vi "Forebrain Main.vi"(8 "error in":errorcluster, 9 "QueueRef":T2, 10 "Mission Notifiers":T1, 11 "NotifierReff":T3) -> (0 "error out":errorcluster)   [LabVIEW 2013]
uses:
  Data/TypeDefs/Notifiers.ctl
  Data/TypeDefs/UTM Location.ctl
  Data/TypeDefs/Sail Set Suggestions.ctl
  Data/TypeDefs/Rudder Set Suggestions.ctl
  Data/TypeDefs/OverrideInformation.ctl
  Data/TypeDefs/OverrideMode.ctl
  Data/TypeDefs/MotorSetup.ctl
  Data/TypeDefs/DynamixelSetupInfo.ctl
  Data/TypeDefs/AirmarStatus.ctl
  Data/TypeDefs/HardwareOnline.ctl
  Data/TypeDefs/DynamixelCycleTracker.ctl
  Data/TypeDefs/RC Input Values.ctl
  Classes/Waypoint/Waypoint.lvclass
  Data/TypeDefs/Queues.ctl
  Data/TypeDefs/MissionNotifiers.ctl
  Classes/Missions/GenericMission/GenericMission.lvclass
  Classes/Obstacle/Obstacle.lvclass
  RIO-OCU_Comm/NetworkStreams/Reader/NetworkStreamReader.lvclass
  RIO-OCU_Comm/NetworkStreams/Writer/NetworkStreamWriter.lvclass
panel:
  out "Number of sailing points added":i32
  out "Added sailing points?":bool
  out "Added intermediate point?":bool
  out "Forebrain Sense Counter":i32
  out "Forebrain Act Loop Counter":i32
  out "Forebrain Think Loop Counter":i32
  out "Connected to OCU?":bool
  # "Debug"
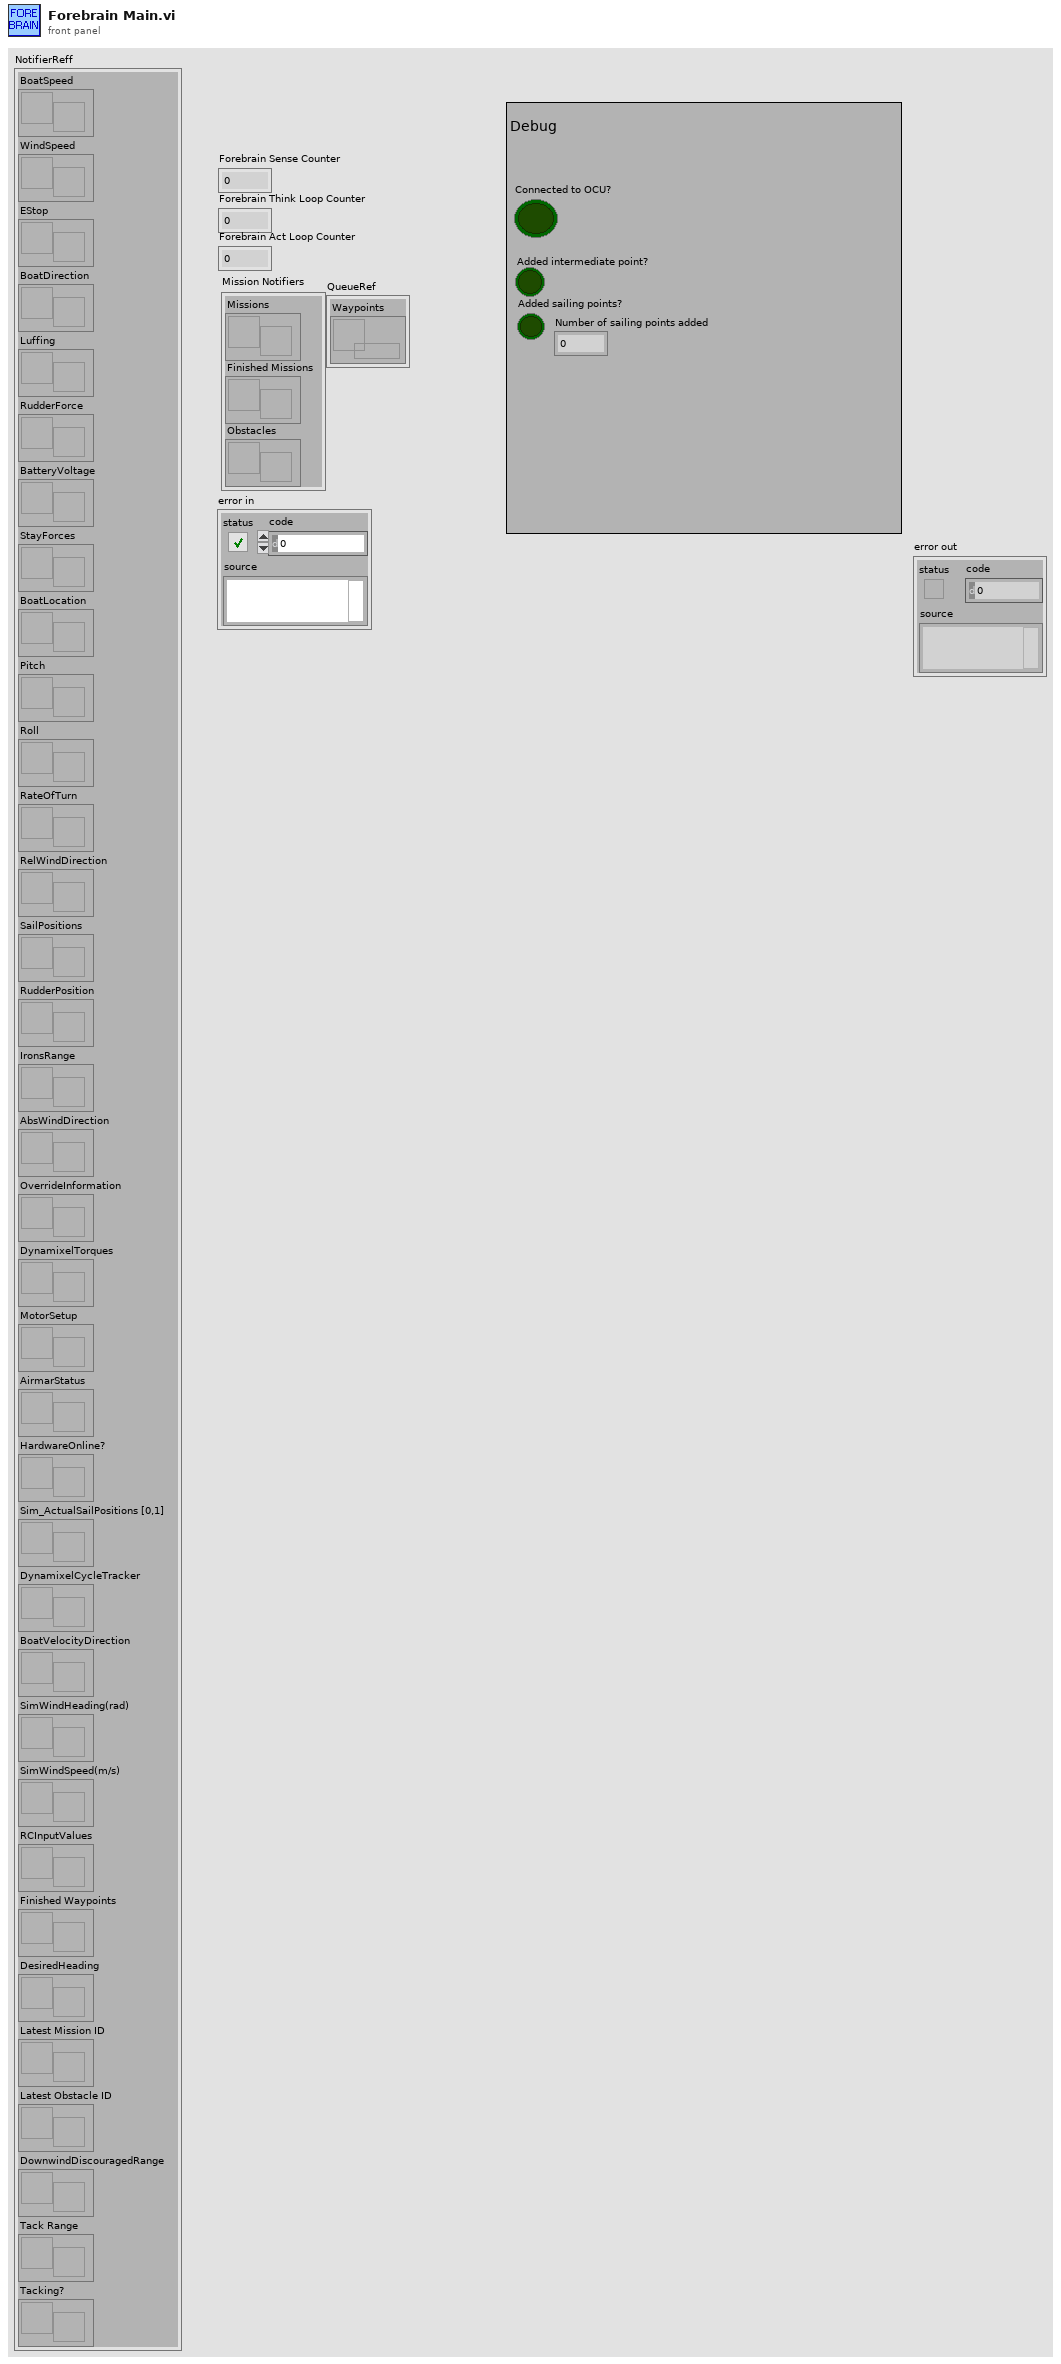
[diagram p1: front panel]
types:
  T1 = typedef "MissionNotifiers.ctl" = cluster{"Missions":refnum<notifier>, "Finished Missions":refnum<notifier>, "Obstacles":refnum<notifier>}
  T2 = typedef "Queues.ctl" = cluster{"Waypoints":refnum<queue>}
  T3 = typedef "Notifiers.ctl" = cluster{"BoatSpeed":refnum<notifier>, "WindSpeed":refnum<notifier>, "EStop":refnum<notifier>, "BoatDirection":refnum<notifier>, "Luffing":refnum<notifier>, "RudderForce":refnum<notifier>, "BatteryVoltage":refnum<notifier>, "StayForces":refnum<notifier>, "BoatLocation":refnum<notifier>, "Pitch":refnum<notifier>, "Roll":refnum<notifier>, "RateOfTurn":refnum<notifier>, "RelWindDirection":refnum<notifier>, "SailPositions":refnum<notifier>, "RudderPosition":refnum<notifier>, "IronsRange":refnum<notifier>, "AbsWindDirection":refnum<notifier>, "OverrideInformation":refnum<notifier>, "DynamixelTorques":refnum<notifier>, "MotorSetup":refnum<notifier>, "AirmarStatus":refnum<notifier>, "HardwareOnline?":refnum<notifier>, "Sim_ActualSailPositions [0,1]":refnum<notifier>, "DynamixelCycleTracker":refnum<notifier>, "BoatVelocityDirection":refnum<notifier>, "SimWindHeading(rad)":refnum<notifier>, "SimWindSpeed(m/s)":refnum<notifier>, "RCInputValues":refnum<notifier>, "Finished Waypoints":refnum<notifier>, "DesiredHeading":refnum<notifier>, "Latest Mission ID":refnum<notifier>, "Latest Obstacle ID":refnum<notifier>, "DownwindDiscouragedRange":refnum<notifier>, "Tack Range":refnum<notifier>, "Tacking?":refnum<notifier>}
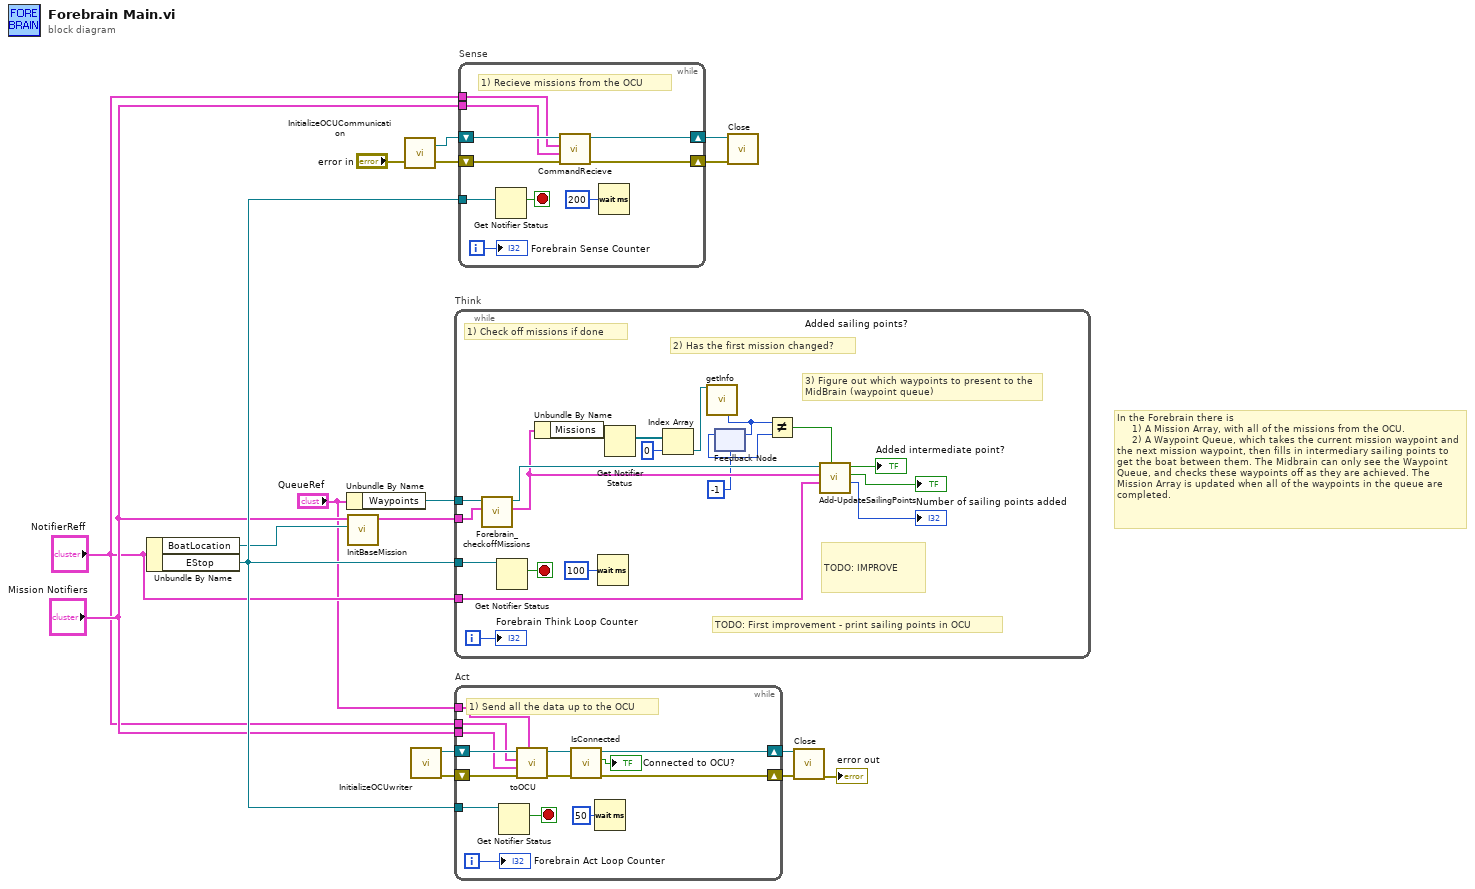
[diagram p0: block diagram]
diagram:
  # "In the Forebrain there is\n     1) A Mission Array, with all of the missions from the OCU.\n     2) A Waypoint Queue, which takes the current mission waypoint and the next mission waypoint, then fills in intermediary sailing points to get the boat between them. The Midbrain can only see the Waypoint Queue, and checks these waypoints off as they are achieved. The Mission Array is updated when all of the waypoints in the queue are completed."
  n1 = Unbundle By Name("NotifierReff") -> ("BoatLocation"=w5:refnum<notifier>, "EStop"=w11:refnum<notifier>)
  n2 = Unbundle By Name("QueueRef") -> ("Waypoints"=w17:refnum<queue>)
  n3 = call "InitBaseMission.vi"("Boat Location"=w5, "Mission Notifiers"="Mission Notifiers") -> ("Mission Notifiers OUT"=w3:T1)  [unwired: 9 in]
  n4 = call "InitializeOCUCommunication.vi"("error in (no error)"="error in") -> ("error out"=w16:errorcluster, "NetworkStreamReader out"=w15:refnum<class "NetworkStreamReader.lvclass">)  [unwired: 1 in]
  n5 = call "InitializeOCUwriter.vi"() -> ("error out"=w8:errorcluster, "NetworkStreamWriter out"=w10:refnum<class "NetworkStreamWriter.lvclass">)  [unwired: 10 in]
  n6 = while "Think" {
    tunnel: w11 -> [w36]
    tunnel: w17 -> [w32]
    tunnel: w3 -> [w33]
    tunnel: "NotifierReff" -> [w21]
    i -> [w34]
    stop <- w37 stop-if-true
    # "TODO: First improvement - print sailing points in OCU"
    # "2) Has the first mission changed?"
    # "TODO: IMPROVE"
    # "3) Figure out which waypoints to present to the MidBrain (waypoint queue)"
    # "1) Check off missions if done"
    n7 = call "Forebrain_checkoffMissions.vi"("Mission Notifiers"=w33, "Waypoints"=w32) -> ("Mission Notifiers OUT"=w30:T1, "Waypoints out"=w31:refnum<queue>)  [unwired: 7 in, 1 out]
    n8 = Get Notifier Status(notifier=w36) -> (current notification=w37:bool)  [unwired: 1 in, 4 out]
    n9 = Unbundle By Name(w30) -> ("Missions"=w29:refnum<notifier>)
    n10 = Wait (ms)(milliseconds to wait=u32 100) -> ()  [unwired: 1 out]
    n11 = Get Notifier Status(notifier=w29) -> (current notification=w28:refnum<class "GenericMission.lvclass">[])  [unwired: 1 in, 4 out]
    n12 = Index Array(array=w28, index=0) -> (element=w26:refnum<class "GenericMission.lvclass">)
    n13 = call-dynamic "getInfo.vi"("GenericMission in"=w26) -> ("ID#"=w25:i16)  [unwired: 6 in, 8 out]
    n14 = feedback-in #1(w25) -> ()
    n15 = feedback #1(i16 -1 ("ID#")) -> (w24:i16)
    n16 = Not Equal?(x=w25, y=w24) -> (x != y?=w22:bool)
    n17 = call "Add-UpdateSailingPoints.vi"("Has the first mission changed?"=w22, "NotifierReff"=w21, "Mission Notifiers"=w30, "Waypoints queue for Midbrain"=w31) -> ("Number of sailing points added"=→"Number of sailing points added":i32, "Added sailing points?"=→"Added sailing points?":bool, "Added intermediate point?"=→"Added intermediate point?":bool)  [unwired: 5 in]
    "Forebrain Think Loop Counter" <- w34
  }
  n18 = while "Act" {
    tunnel: w11 -> [w50]
    shift-right: [w43] -> w9
    shift-left: w10 -> [w49]
    shift-right: [w44] -> w7
    shift-left: w8 -> [w48]
    tunnel: "NotifierReff" -> [w47]
    tunnel: "Mission Notifiers" -> [w39]
    tunnel: "QueueRef" -> [w38]
    i -> [w41]
    stop <- w40 stop-if-true
    # "1) Send all the data up to the OCU"
    n19 = Get Notifier Status(notifier=w50) -> (current notification=w40:bool)  [unwired: 1 in, 4 out]
    n20 = call "toOCU.vi"("QueueRef"=w38, "error in (no error)"=w48, "Mission Notifiers"=w39, "NotifierReff"=w47, "NetworkStreamWriter in"=w49) -> ("error out"=w46:errorcluster, "NetworkStreamWriter out"=w45:refnum<class "NetworkStreamWriter.lvclass">)  [unwired: 5 in]
    n21 = call "IsConnected.vi"("error in (no error)"=w46, "NetworkStreamWriter in"=w45) -> ("error out"=w44:errorcluster, "Connected?"=→"Connected to OCU?":bool, "NetworkStreamWriter out"=w43:refnum<class "NetworkStreamWriter.lvclass">)  [unwired: 7 in]
    n22 = Wait (ms)(milliseconds to wait=u32 50) -> ()  [unwired: 1 out]
    "Forebrain Act Loop Counter" <- w41
  }
  n23 = while "Sense" {
    tunnel: w11 -> [w60]
    shift-right: [w58] -> w14
    shift-left: w16 -> [w59]
    shift-right: [w54] -> w13
    shift-left: w15 -> [w56]
    tunnel: "NotifierReff" -> [w55]
    tunnel: "Mission Notifiers" -> [w52]
    i -> [w53]
    stop <- w61 stop-if-true
    # "1) Recieve missions from the OCU"
    n24 = Get Notifier Status(notifier=w60) -> (current notification=w61:bool)  [unwired: 1 in, 4 out]
    n25 = call "CommandRecieve.vi"("error in (no error)"=w59, "Mission Notifiers"=w52, "NotifierReff"=w55, "NetworkStreamReader in"=w56) -> ("error out"=w58:errorcluster, "NetworkStreamReader out"=w54:refnum<class "NetworkStreamReader.lvclass">)  [unwired: 6 in]
    n26 = Wait (ms)(milliseconds to wait=u32 200) -> ()  [unwired: 1 out]
    "Forebrain Sense Counter" <- w53
  }
  n27 = call "Close.vi"("error in (no error)"=w14, "NetworkStreamReader in"=w13) -> ()  [unwired: 9 in, 1 out]
  n28 = call "Close.vi"("error in (no error)"=w7, "NetworkStreamWriter in"=w9) -> ("error out"=→"error out":errorcluster)  [unwired: 9 in]
